vi "send_request.vi"(0 "connection ID":refnum<k5>, 1 "timeout ms":i32, 2 "function name":string, 3 "args":variant, 4 "kwargs":variant, 5 "error in":errorcluster, 6 "Service name":string) -> (14 "connection ID out":refnum<k5>, 15 "#bytes written":i32, 16 "bytes":string, 19 "error out":errorcluster)   [LabVIEW 2010]
uses:
  i3-json-1.0.0-10/i3-json.lvlib
  i3-json-1.0.0-10/JSON Generation/Create Value Files/Create Value - Object.vi
  i3-json-1.0.0-10/JSON Generation/Add Object Parameter Files/Add Object Parameter - String.vi
  i3-json-1.0.0-10/JSON Generation/Add Object Parameter Files/Add Object Parameter - Boolean.vi
  i3-json-1.0.0-10/JSON Generation/Add Object Parameter Files/Add Object Parameter - Array.vi
  i3-json-1.0.0-10/JSON Generation/Add Object Parameter Files/Add Object Parameter - Object.vi
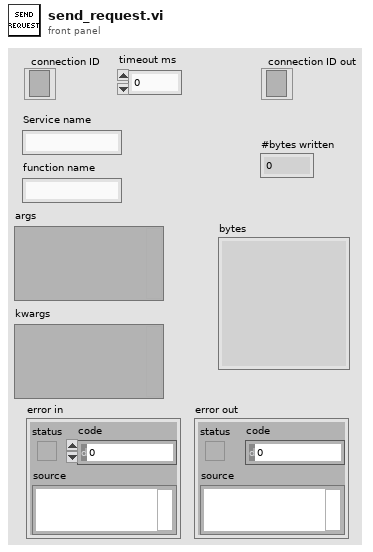
[diagram p1: front panel]
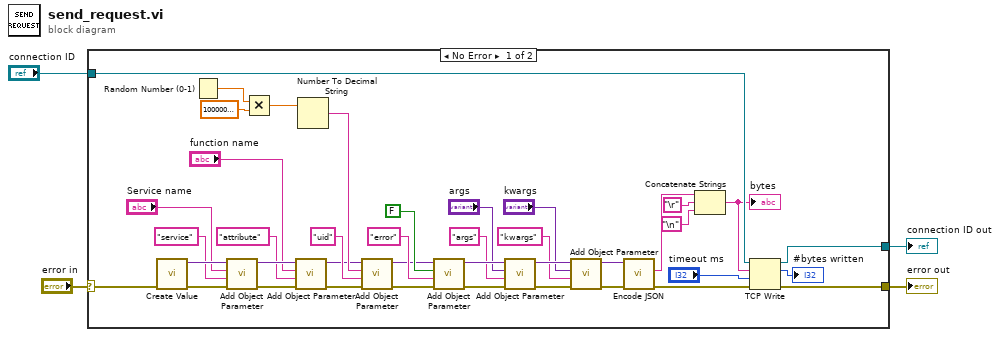
[diagram p0: block diagram]
diagram:
  n1 = case shown="No Error" "error in" {
    selector: "error in" -> [w29 w46]
    tunnel: "connection ID" -> [w43 w45]
    tunnel: [w42 w46] -> w3
    tunnel: [w40 w45] -> w2
    frame No Error {
      n2 = call-poly "Create Value.vi"("error in (no error)"=w29) -> ("error out"=w28:errorcluster, "JSON Tree"=w35:variant)  [unwired: 9 in]
      n3 = Random Number (0-1)() -> (number: 0 to 1=w26:dbl)
      n4 = call-poly "Add Object Parameter.vi"("error in (no error)"=w28, "Name"="service" ("Default Value if JSON Null"), "String"="Service name", "JSON Tree in (JSON Object)"=w35) -> ("error out"=w19:errorcluster, "JSON Tree out (JSON Object)"=w22:variant)  [unwired: 6 in]
      n5 = Multiply(x=w26, y=1000000000000.0) -> (x*y=w24:dbl)
      n6 = call-poly "Add Object Parameter.vi"("error in (no error)"=w19, "Name"="attribute" ("Default Value if JSON Null"), "String"="function name", "JSON Tree in (JSON Object)"=w22) -> ("error out"=w18:errorcluster, "JSON Tree out (JSON Object)"=w17:variant)  [unwired: 6 in]
      n7 = Number To Decimal String(number=w24) -> (decimal integer string=w23:string)  [unwired: 1 in]
      n8 = call-poly "Add Object Parameter.vi"("error in (no error)"=w18, "Name"="uid" ("name"), "String"=w23, "JSON Tree in (JSON Object)"=w17) -> ("error out"=w14:errorcluster, "JSON Tree out (JSON Object)"=w15:variant)  [unwired: 6 in]
      n9 = call-poly "Add Object Parameter.vi"("error in (no error)"=w14, "Name"="error", "Boolean"=FALSE, "JSON Tree in (JSON Object)"=w15) -> ("error out"=w16:errorcluster, "JSON Tree out (JSON Object)"=w13:variant)  [unwired: 6 in]
      n10 = call-poly "Add Object Parameter.vi"("error in (no error)"=w16, "Name"="args", "JSON Array"="args", "JSON Tree in (JSON Object)"=w13) -> ("error out"=w7:errorcluster, "JSON Tree out (JSON Object)"=w10:variant)  [unwired: 6 in]
      n11 = call-poly "Add Object Parameter.vi"("error in (no error)"=w7, "Name"="kwargs", "JSON Object"="kwargs", "JSON Tree in (JSON Object)"=w10) -> ("error out"=w8:errorcluster, "JSON Tree out (JSON Object)"=w9:variant)  [unwired: 6 in]
      n12 = call "Encode JSON.vi"("error in (no error)"=w8, "JSON Tree"=w9) -> ("error out"=w33:errorcluster, "String"=w39:string)  [unwired: 4 in]
      n13 = Concatenate Strings(w39, "\r", "\n") -> (w36:string)
      "bytes" <- w36
      n14 = TCP Write(connection ID=w43, data in=w36, error in (no error)=w33, 9:"timeout ms") -> (connection ID out=w40:refnum<k5>, bytes written=→"#bytes written":i32, error out=w42:errorcluster)
    }
    frame Error {
    }
  }
  "error out" <- w3
  "connection ID out" <- w2
